vi "parse config data from file.vi"(7 "Calibration Config":T1, 8 "Error in":errorcluster caption="Error in (no error)", 11 "Array":cluster{"String":string, string[]}[](array[cluster])) -> (0 "Error out":errorcluster, 3 "Config cluster":T1)   [LabVIEW 2020]
uses:
  Typedefs/Calibration config.ctl
  Typedefs/Objective Config.ctl
  Typedefs/Prechirper Cal Config.ctl
  Typedefs/PreChirper constants.ctl
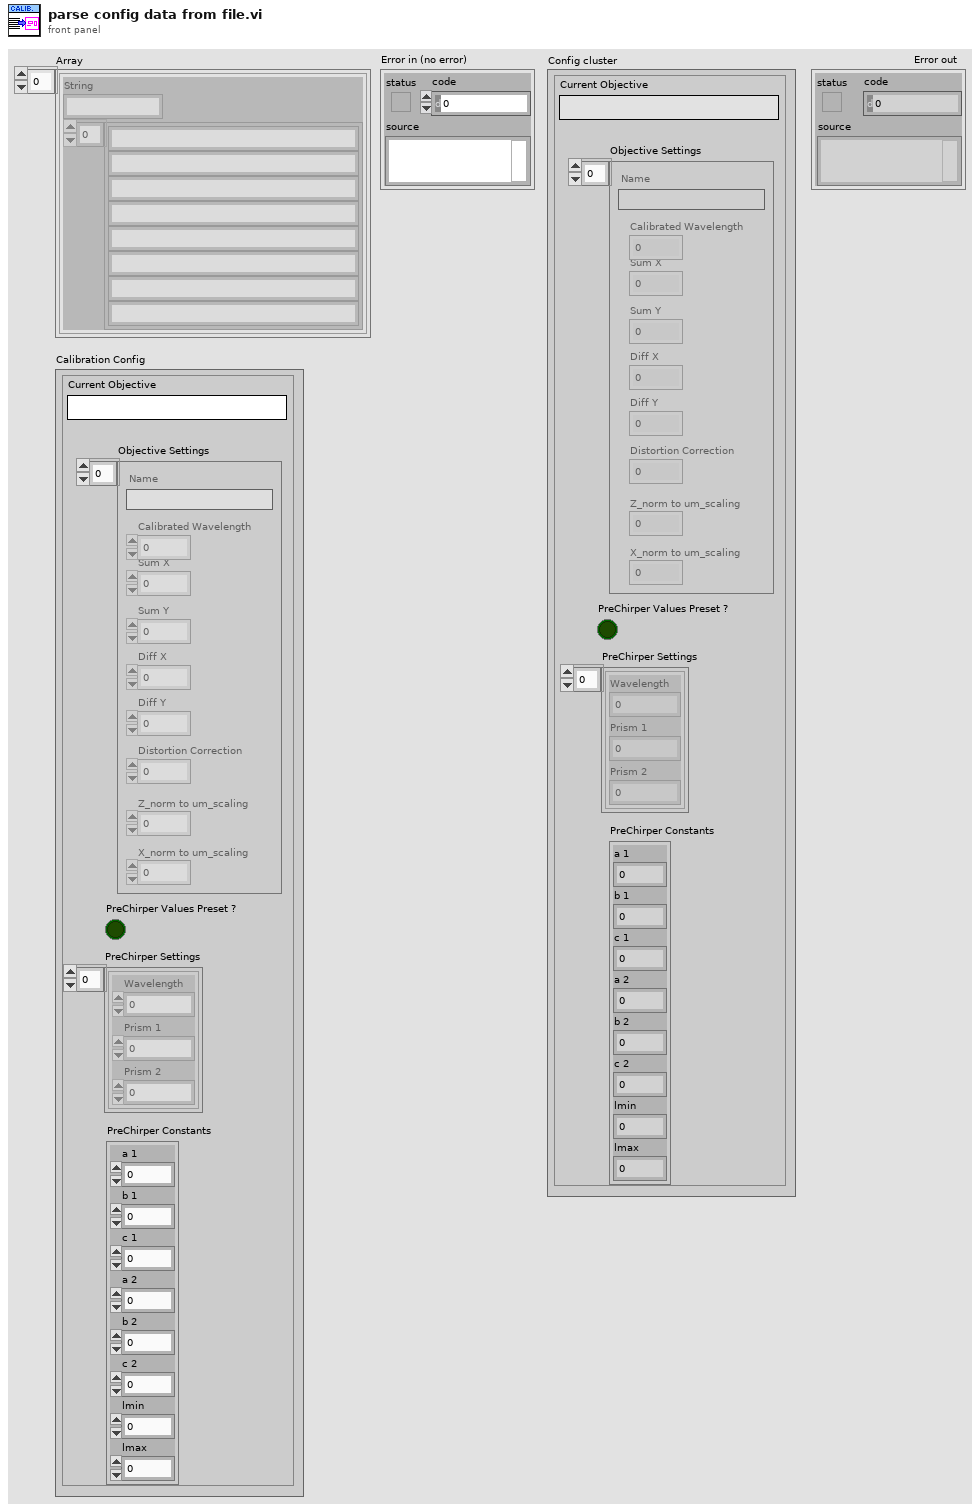
[diagram p1: front panel]
types:
  T1 = typedef "Calibration config.ctl" = cluster{"Current Objective":string, "Objective Settings":T2[], "PreChirper Values Preset ?":bool, "PreChirper Settings":T3[], "PreChirper Constants":T4}
  T2 = typedef "Objective Config.ctl" = cluster{"Name":string, "Sum X":dbl, "Sum Y":dbl, "Diff X":dbl, "Diff Y":dbl, "Distortion Correction":dbl, "Z_norm to um_scaling":dbl, "X_norm to um_scaling":dbl, "Calibrated Wavelength":dbl}
  T3 = typedef "Prechirper Cal Config.ctl" = cluster{"Wavelength":i32, "Prism 1":i32, "Prism 2":i32}
  T4 = typedef "PreChirper constants.ctl" = cluster{"a 1":i32, "b 1":i32, "c 1":i32, "a 2":i32, "b 2":i32, "c 2":i32, "lmin":i32, "lmax":i32}
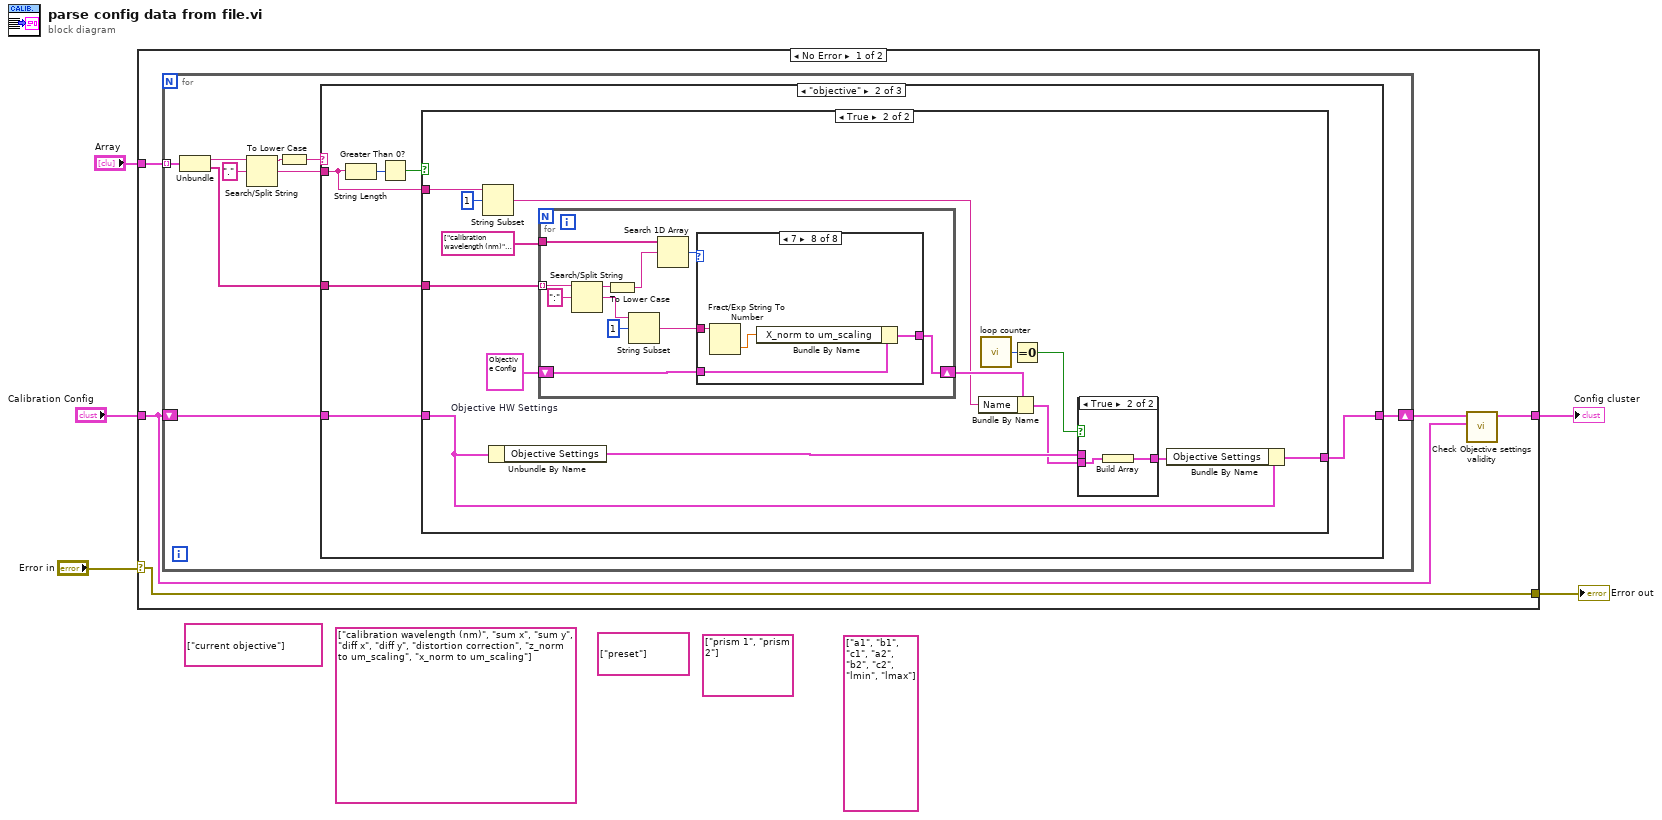
[diagram p0: block diagram]
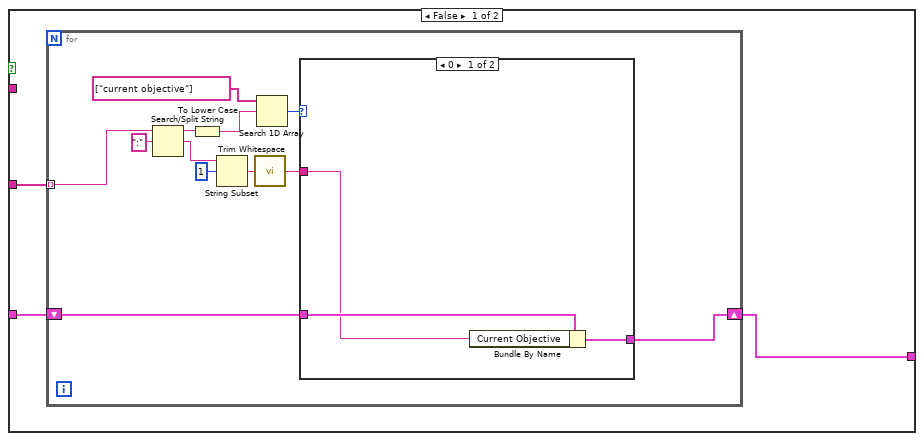
[diagram p3: hidden frame]
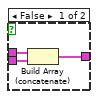
[diagram p5: hidden frame]
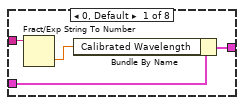
[diagram p6: hidden frame]
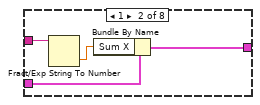
[diagram p7: hidden frame]
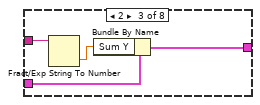
[diagram p8: hidden frame]
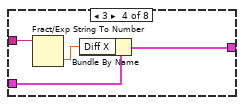
[diagram p9: hidden frame]
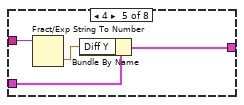
[diagram p10: hidden frame]
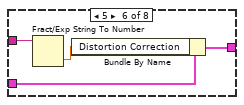
[diagram p11: hidden frame]
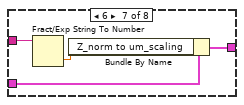
[diagram p12: hidden frame]
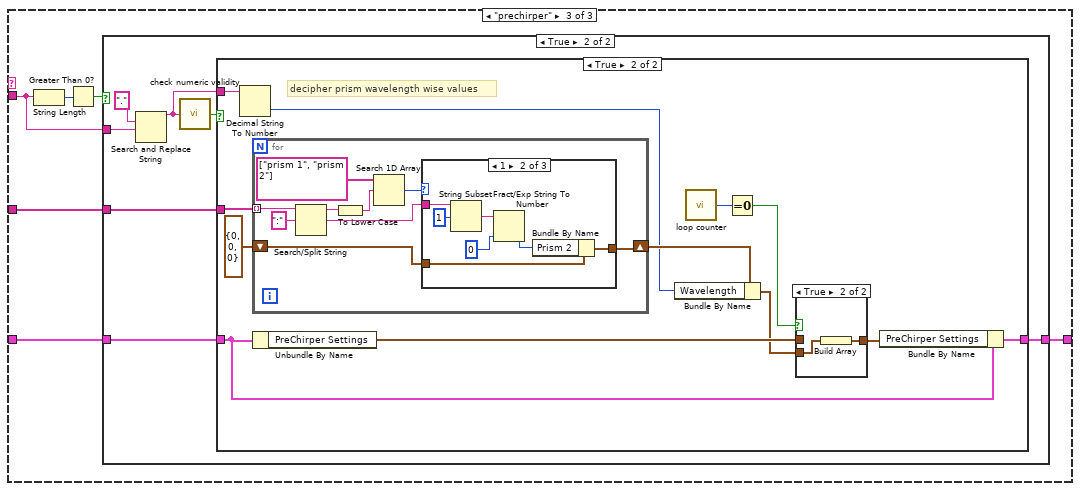
[diagram p13: hidden frame]
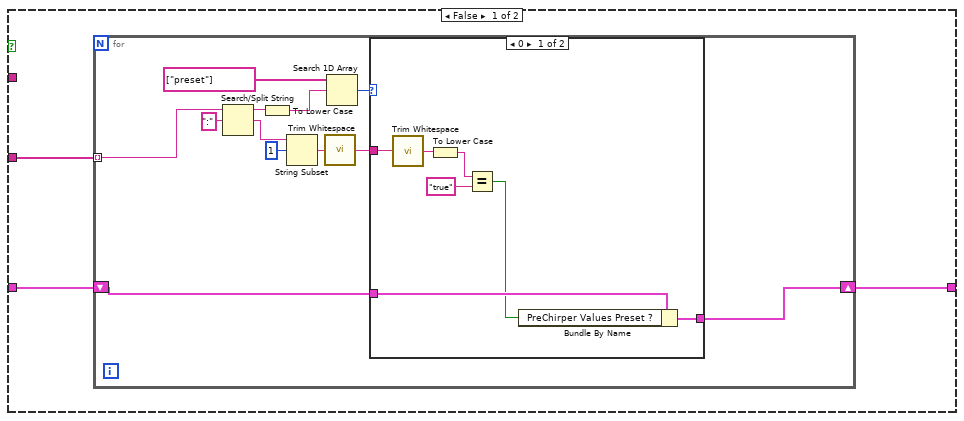
[diagram p14: hidden frame]
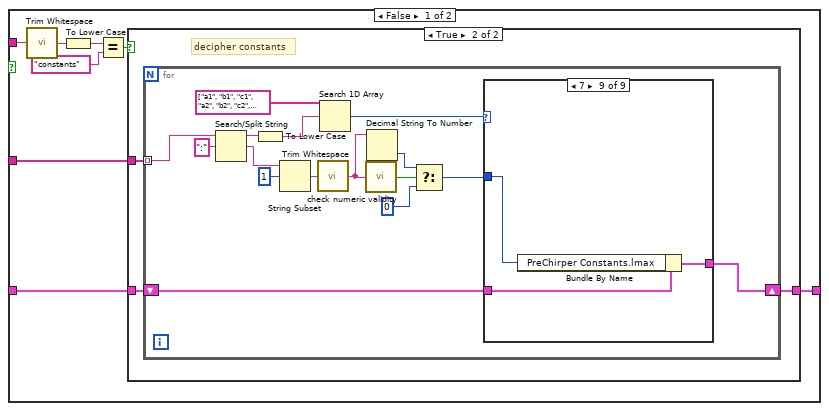
[diagram p16: hidden frame]
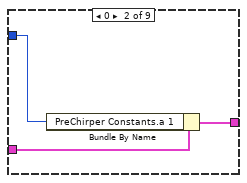
[diagram p19: hidden frame]
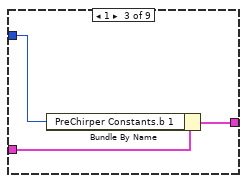
[diagram p20: hidden frame]
diagram:
  (unwired) string[] ["a1", "b1", "c1", "a2", "b2", "c2", "lmin", "lmax"]
  (unwired) string[] ["preset"]
  (unwired) string[] ["prism 1", "prism 2"]
  (unwired) string[] ["calibration wavelength (nm)", "sum x", "sum y", "diff x", "diff y", "distortion correction", "z_norm to um_scaling", "x_norm to um_scaling"]
  (unwired) string[] ["current objective"]
  n1 = case shown="No Error" "Error in" {
    selector: "Error in" -> [w9 w239]
    tunnel: "Array" -> [w10 _]
    tunnel: "Calibration Config" -> [w7 w238]
    tunnel: [w6 w238] -> w1
    tunnel: [w9 w239] -> w2
    frame No Error {
      n2 = for {
        tunnel: w10 -> [w19] mode=indexing
        shift-right: [w12] -> w8
        shift-left: w7 -> [w13]
        n3 = Unbundle(w19) -> ("String"=w17:string, w18:string[])
        n4 = Search/Split String(string=w17, search string/char (-)="." ("regular expression")) -> (substring before match=w15:string, match + rest of string=w14:string)  [unwired: 1 in, 1 out]
        n5 = To Lower Case(string=w15) -> (all lower case string=w11:string)
        n6 = case shown="\"objective\"" w11 {
          tunnel: w18 -> [_ w21 w111]
          tunnel: w14 -> [_ w24 w110]
          tunnel: w13 -> [w20 w23 w109]
          tunnel: [w20 w22 w108] -> w12
          frame Default {
          }
          frame "objective" {
            n7 = String Length(string=w24) -> (length=w26:i32)
            n8 = Greater Than 0?(x=w26) -> (x > 0?=w25:bool)
            n9 = case shown="True" w25 {
              tunnel: w24 -> [_ w49]
              tunnel: w23 -> [w29 w53]
              tunnel: [w28 w51] -> w22
              tunnel: w21 -> [w27 w59]
              frame False {
                n10 = for {
                  shift-right: [w31] -> w28
                  shift-left: w29 -> [w32]
                  tunnel: w27 -> [w30] mode=indexing
                  n11 = Search/Split String(string=w30, search string/char (-)=":") -> (substring before match=w40:string, match + rest of string=w37:string)  [unwired: 1 in, 1 out]
                  n12 = To Lower Case(string=w40) -> (all lower case string=w39:string)
                  n13 = String Subset(string=w37, offset (0)=1) -> (substring=w35:string)  [unwired: 1 in]
                  n14 = call <vilib>:"Trim Whitespace.vi"("string"=w35) -> ("trimmed string"=w33:string)  [unwired: 1 in]
                  n15 = Search 1D Array(1D array=string[] ["current objective"], element=w39) -> (index of element=w34:i32)  [unwired: 1 in]
                  n16 = case shown="0" w34 {
                    tunnel: w33 -> [w43 _]
                    tunnel: w32 -> [w44 w45]
                    tunnel: [w42 w45] -> w31
                    frame 0 {
                      n17 = Bundle By Name(cluster=w44, "Current Objective"=w43) -> (w42:T1)
                    }
                    frame -1, Default {
                    }
                  }
                }
              }
              frame True {
                w58 = T2 {"Name"="", "Sum X"=0.0, "Sum Y"=0.0, "Diff X"=0.0, "Diff Y"=0.0, "Distortion Correction"=0.0, "Z_norm to um_scaling"=0.0, "X_norm to um_scaling"=0.0, "Calibrated Wavelength"=0.0}  # Objective HW Settings
                n18 = String Subset(string=w49, offset (0)=1) -> (substring=w48:string)  [unwired: 1 in]
                n19 = Unbundle By Name(w53) -> ("Objective Settings"=w55:T2[])
                n20 = for {
                  tunnel: string[] ["calibration wavelength (nm)", "sum x", "sum y", "diff x", "diff y", "distortion correction", "z_norm to um_scaling", "x_norm to um_scaling"] -> [w75]
                  tunnel: w59 -> [w70] mode=indexing
                  shift-right: [w65] -> w56
                  shift-left: w58 -> [w73]
                  n21 = Search/Split String(string=w70, search string/char (-)=":") -> (substring before match=w71:string, match + rest of string=w68:string)  [unwired: 1 in, 1 out]
                  n22 = To Lower Case(string=w71) -> (all lower case string=w69:string)
                  n23 = String Subset(string=w68, offset (0)=1) -> (substring=w66:string)  [unwired: 1 in]
                  n24 = Search 1D Array(1D array=w75, element=w69) -> (index of element=w74:i32)  [unwired: 1 in]
                  n25 = case shown="7" w74 {
                    tunnel: w73 -> [w79 w83 w87 w91 w95 w99 w103 w107]
                    tunnel: w66 -> [w78 w82 w86 w90 w94 w98 w102 w106]
                    tunnel: [w76 w80 w84 w88 w92 w96 w100 w104] -> w65
                    frame 0, Default {
                      n26 = Fract/Exp String To Number(string=w78) -> (number=w77:dbl)  [unwired: 3 in, 1 out]
                      n27 = Bundle By Name(cluster=w79, "Calibrated Wavelength"=w77) -> (w76:T2)
                    }
                    frame 1 {
                      n28 = Fract/Exp String To Number(string=w82) -> (number=w81:dbl)  [unwired: 3 in, 1 out]
                      n29 = Bundle By Name(cluster=w83, "Sum X"=w81) -> (w80:T2)
                    }
                    frame 2 {
                      n30 = Fract/Exp String To Number(string=w86) -> (number=w85:dbl)  [unwired: 3 in, 1 out]
                      n31 = Bundle By Name(cluster=w87, "Sum Y"=w85) -> (w84:T2)
                    }
                    frame 3 {
                      n32 = Fract/Exp String To Number(string=w90) -> (number=w89:dbl)  [unwired: 3 in, 1 out]
                      n33 = Bundle By Name(cluster=w91, "Diff X"=w89) -> (w88:T2)
                    }
                    frame 4 {
                      n34 = Fract/Exp String To Number(string=w94) -> (number=w93:dbl)  [unwired: 3 in, 1 out]
                      n35 = Bundle By Name(cluster=w95, "Diff Y"=w93) -> (w92:T2)
                    }
                    frame 5 {
                      n36 = Fract/Exp String To Number(string=w98) -> (number=w97:dbl)  [unwired: 3 in, 1 out]
                      n37 = Bundle By Name(cluster=w99, "Distortion Correction"=w97) -> (w96:T2)
                    }
                    frame 6 {
                      n38 = Fract/Exp String To Number(string=w102) -> (number=w101:dbl)  [unwired: 3 in, 1 out]
                      n39 = Bundle By Name(cluster=w103, "Z_norm to um_scaling"=w101) -> (w100:T2)
                    }
                    frame 7 {
                      n40 = Fract/Exp String To Number(string=w106) -> (number=w105:dbl)  [unwired: 3 in, 1 out]
                      n41 = Bundle By Name(cluster=w107, "X_norm to um_scaling"=w105) -> (w104:T2)
                    }
                  }
                }
                n42 = Bundle By Name(cluster=w56, "Name"=w48) -> (w54:T2)
                n43 = call "loop counter.vi"() -> ("Count"=w47:i32)  [unwired: 9 in]
                n44 = Equal To 0?(x=w47) -> (x = 0?=w46:bool)
                n45 = case shown="True" w46 {
                  tunnel: w55 -> [w62 _]
                  tunnel: w54 -> [w61 w64]
                  tunnel: [w60 w63] -> w52
                  frame False {
                    n46 = Build Array (concatenate)(w62, w61) -> (w60:T2[])
                  }
                  frame True {
                    n47 = Build Array(w64) -> (w63:T2[])
                  }
                }
                n48 = Bundle By Name(cluster=w53, "Objective Settings"=w52) -> (w51:T1)
              }
            }
          }
          frame "prechirper" {
            n49 = String Length(string=w110) -> (length=w113:i32)
            n50 = Greater Than 0?(x=w113) -> (x > 0?=w112:bool)
            n51 = case shown="True" w112 {
              tunnel: w111 -> [w115 w139]
              tunnel: w110 -> [_ w143]
              tunnel: w109 -> [w116 w138]
              tunnel: [w114 w137] -> w108
              frame False {
                n52 = for {
                  tunnel: w115 -> [w118] mode=indexing
                  shift-right: [w119] -> w114
                  shift-left: w116 -> [w120]
                  n53 = Search/Split String(string=w118, search string/char (-)=":") -> (substring before match=w127:string, match + rest of string=w125:string)  [unwired: 1 in, 1 out]
                  n54 = To Lower Case(string=w127) -> (all lower case string=w126:string)
                  n55 = String Subset(string=w125, offset (0)=1) -> (substring=w123:string)  [unwired: 1 in]
                  n56 = call <vilib>:"Trim Whitespace.vi"("string"=w123) -> ("trimmed string"=w121:string)  [unwired: 1 in]
                  n57 = Search 1D Array(1D array=string[] ["preset"], element=w126) -> (index of element=w122:i32)  [unwired: 1 in]
                  n58 = case shown="0" w122 {
                    tunnel: w121 -> [w133 _]
                    tunnel: w120 -> [w135 w136]
                    tunnel: [w134 w136] -> w119
                    frame 0 {
                      n59 = call <vilib>:"Trim Whitespace.vi"("string"=w133) -> ("trimmed string"=w132:string)  [unwired: 1 in]
                      n60 = To Lower Case(string=w132) -> (all lower case string=w131:string)
                      n61 = Equal?(x=w131, y="true") -> (x = y?=w129:bool)
                      n62 = Bundle By Name(cluster=w135, "PreChirper Values Preset ?"=w129) -> (w134:T1)
                    }
                    frame -1, Default {
                    }
                  }
                }
              }
              frame True {
                n63 = Search and Replace String(input string=w143, search string=".") -> (result string=w140:string)  [unwired: 6 in, 3 out]
                n64 = call "check numeric validity.vi"("Numeric string"=w140) -> ("Valid ?"=w141:bool)  [unwired: 8 in]
                n65 = case shown="True" w141 {
                  tunnel: w140 -> [w151 w208]
                  tunnel: w139 -> [w144 w207]
                  tunnel: w138 -> [w146 w201]
                  tunnel: [w145 w199] -> w137
                  frame False {
                    n66 = call <vilib>:"Trim Whitespace.vi"("string"=w151) -> ("trimmed string"=w150:string)  [unwired: 1 in]
                    n67 = To Lower Case(string=w150) -> (all lower case string=w149:string)
                    n68 = Equal?(x=w149, y="constants") -> (x = y?=w147:bool)
                    n69 = case shown="True" w147 {
                      tunnel: w146 -> [w152 w155]
                      tunnel: [w152 w153] -> w145
                      tunnel: w144 -> [_ w154]
                      frame False {
                        # "nothing found, hence empty"
                      }
                      frame True {
                        # "decipher constants"
                        n70 = for {
                          shift-right: [w159] -> w153
                          shift-left: w155 -> [w171]
                          tunnel: w154 -> [w164] mode=indexing
                          n71 = Search/Split String(string=w164, search string/char (-)=":") -> (substring before match=w169:string, match + rest of string=w167:string)  [unwired: 1 in, 1 out]
                          n72 = To Lower Case(string=w169) -> (all lower case string=w168:string)
                          n73 = String Subset(string=w167, offset (0)=1) -> (substring=w165:string)  [unwired: 1 in]
                          n74 = call <vilib>:"Trim Whitespace.vi"("string"=w165) -> ("trimmed string"=w161:string)  [unwired: 1 in]
                          n75 = Search 1D Array(1D array=string[] ["a1", "b1", "c1", "a2", "b2", "c2", "lmin", "lmax"], element=w168) -> (index of element=w163:i32)  [unwired: 1 in]
                          n76 = call "check numeric validity.vi"("Numeric string"=w161) -> ("Valid ?"=w162:bool)  [unwired: 8 in]
                          n77 = Decimal String To Number(string=w161) -> (number=w157:i32)  [unwired: 2 in, 1 out]
                          n78 = Select(t=w157, s=w162, f=0 ("t")) -> (s? t:f=w160:i32)
                          n79 = case shown="7" w163 {
                            tunnel: w171 -> [w172 w175 w178 w181 w184 w187 w190 w193 w196]
                            tunnel: w160 -> [_ w174 w177 w180 w183 w186 w189 w192 w195]
                            tunnel: [w172 w173 w176 w179 w182 w185 w188 w191 w194] -> w159
                            frame -1, Default {
                            }
                            frame 0 {
                              n80 = Bundle By Name(cluster=w175, "PreChirper Constants.a 1"=w174) -> (w173:T1)
                            }
                            frame 1 {
                              n81 = Bundle By Name(cluster=w178, "PreChirper Constants.b 1"=w177) -> (w176:T1)
                            }
                            frame 2 {
                              n82 = Bundle By Name(cluster=w181, "PreChirper Constants.c 1"=w180) -> (w179:T1)
                            }
                            frame 3 {
                              n83 = Bundle By Name(cluster=w184, "PreChirper Constants.a 2"=w183) -> (w182:T1)
                            }
                            frame 4 {
                              n84 = Bundle By Name(cluster=w187, "PreChirper Constants.b 2"=w186) -> (w185:T1)
                            }
                            frame 5 {
                              n85 = Bundle By Name(cluster=w190, "PreChirper Constants.c 2"=w189) -> (w188:T1)
                            }
                            frame 6 {
                              n86 = Bundle By Name(cluster=w193, "PreChirper Constants.lmin"=w192) -> (w191:T1)
                            }
                            frame 7 {
                              n87 = Bundle By Name(cluster=w196, "PreChirper Constants.lmax"=w195) -> (w194:T1)
                            }
                          }
                        }
                      }
                    }
                  }
                  frame True {
                    # "decipher prism wavelength wise values"
                    n88 = Decimal String To Number(string=w208) -> (number=w204:i32)  [unwired: 2 in, 1 out]
                    n89 = for {
                      tunnel: w207 -> [w222] mode=indexing
                      shift-right: [w214] -> w205
                      shift-left: T3 {"Wavelength"=0, "Prism 1"=0, "Prism 2"=0} ("Prechirper Cal Config") -> [w216]
                      n90 = Search/Split String(string=w222, search string/char (-)=":") -> (substring before match=w219:string, match + rest of string=w215:string)  [unwired: 1 in, 1 out]
                      n91 = To Lower Case(string=w219) -> (all lower case string=w218:string)
                      n92 = Search 1D Array(1D array=string[] ["prism 1", "prism 2"], element=w218) -> (index of element=w217:i32)  [unwired: 1 in]
                      n93 = case shown="1" w217 {
                        tunnel: w216 -> [w229 w236 w237]
                        tunnel: w215 -> [w227 w234 _]
                        tunnel: [w224 w231 w237] -> w214
                        frame 0 {
                          n94 = String Subset(string=w227, offset (0)=1) -> (substring=w226:string)  [unwired: 1 in]
                          n95 = Fract/Exp String To Number(string=w226, default (0 dbl)=0) -> (number=w225:i32)  [unwired: 2 in, 1 out]
                          n96 = Bundle By Name(cluster=w229, "Prism 1"=w225) -> (w224:T3)
                        }
                        frame 1 {
                          n97 = String Subset(string=w234, offset (0)=1) -> (substring=w233:string)  [unwired: 1 in]
                          n98 = Fract/Exp String To Number(string=w233, default (0 dbl)=0) -> (number=w232:i32)  [unwired: 2 in, 1 out]
                          n99 = Bundle By Name(cluster=w236, "Prism 2"=w232) -> (w231:T3)
                        }
                        frame -1, Default {
                        }
                      }
                    }
                    n100 = Unbundle By Name(w201) -> ("PreChirper Settings"=w203:T3[])
                    n101 = Bundle By Name(cluster=w205, "Wavelength"=w204) -> (w202:T3)
                    n102 = call "loop counter.vi"() -> ("Count"=w198:i32)  [unwired: 9 in]
                    n103 = Equal To 0?(x=w198) -> (x = 0?=w197:bool)
                    n104 = case shown="True" w197 {
                      tunnel: w203 -> [w211 _]
                      tunnel: w202 -> [w210 w213]
                      tunnel: [w209 w212] -> w200
                      frame False {
                        n105 = Build Array (concatenate)(w211, w210) -> (w209:T3[])
                      }
                      frame True {
                        n106 = Build Array(w213) -> (w212:T3[])
                      }
                    }
                    n107 = Bundle By Name(cluster=w201, "PreChirper Settings"=w200) -> (w199:T1)
                  }
                }
              }
            }
          }
        }
      }
      n108 = call "Check Objective settings validity.vi"("Default Calibration"=w7, "Loaded \nCalibration Config"=w8) -> ("Loaded \nCalibration Config"=w6:T1)  [unwired: 9 in]
    }
    frame Error {
    }
  }
  "Config cluster" <- w1
  "Error out" <- w2
